vi "Actor Core.vi"(8 "error in":errorcluster, 11 "Timed Loop Controller":refnum<class "Timed Loop Controller.lvclass">) -> (0 "error out":errorcluster, 3 "Actor out":refnum<class "Actor.lvclass">)   [LabVIEW 2016, in "Timed Loop Controller.lvlib" / "Timed Loop Controller.lvclass"]
doc: "This is Actor Core.vi, the main message handling loop for Actors. An actor usually just sits in this loop and processes messages as they arrive. Any error returned by the message Do.vi call will stop the loop, with error code 43 as the cannonical signal to stop with no error sent to caller. Descendants may override that in Handle Error.vi."
uses:
  Timed Loop Controller.lvclass
  C:/Program Files (x86)/National Instruments/LabVIEW 2016/vi.lib/ActorFramework/Actor/Actor.lvclass
  <vilib>/ActorFramework/Actor/Actor.lvclass
  <vilib>/ActorFramework/Actor/Actor.lvclass/Actor.ctl
  <vilib>/ActorFramework/Message Enqueuer/Message Enqueuer.lvclass/Message Enqueuer.ctl
  Timed Loop Controller.lvclass/Timed Loop Controller.ctl
  <vilib>/ActorFramework/Message Enqueuer/Init from Existing Queue.vi
  <vilib>/ActorFramework/Message Enqueuer/Enqueue.vi
  Timed Loop Controller Messages/Update Msg/Update Msg.lvclass
  C:/Program Files (x86)/National Instruments/LabVIEW 2016/vi.lib/ActorFramework/Message/Message.lvclass
  <vilib>/Utility/LVClass/Get LV Class Name.vi
  <resource>/AFDebug/Generate Trace for Message.vi
  <vilib>/ActorFramework/Message Priority Queue/Priority Enqueue.vi
  Controller Actor/Controller Actor.lvclass
  <vilib>/ActorFramework/Message Enqueuer/Message Enqueuer.lvclass
panel:
  in  "stop?":bool
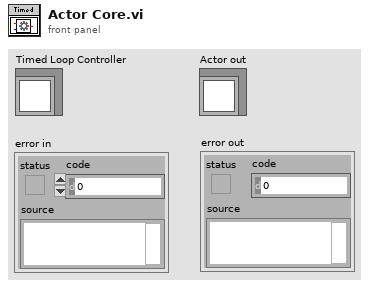
[diagram p1: front panel]
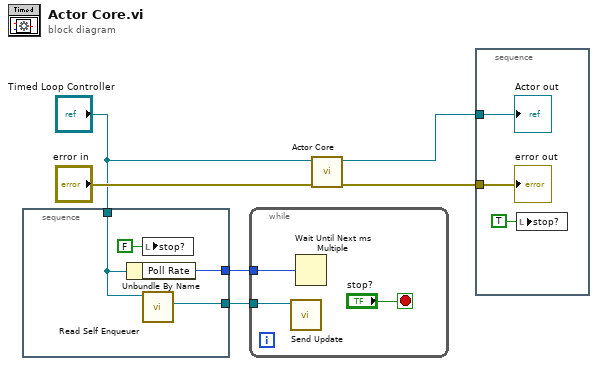
[diagram p0: block diagram]
diagram:
  n1 = stacked-sequence {
    tunnel: "Timed Loop Controller" -> [w10]
    tunnel: [w9] -> w2
    tunnel: [w8] -> w1
    frame #0 {
      n2 = Unbundle By Name(w10) -> ("Poll Rate"=w9:u32)
      n3 = local write "stop?"(FALSE) -> ()
      n4 = call <vilib>:"Read Self Enqueuer.vi"("Actor"=w10) -> ("Self Enqueuer"=w8:refnum<class "Message Enqueuer.lvclass">)  [unwired: 10 in]
    }
  }
  n5 = while {
    tunnel: w1 -> [w13]
    tunnel: w2 -> [w11]
    stop <- "stop?" stop-if-true
    n6 = call "Send Update.vi"("Message Enqueuer in"=w13) -> ()  [unwired: 9 in, 2 out]
    n7 = Wait Until Next ms Multiple(millisecond multiple=w11) -> ()  [unwired: 1 out]
  }
  n8 = call-parent "Actor Core.vi"("error in"="error in", "Event Source in"="Timed Loop Controller") -> ("error out"=w6:errorcluster, "Event Source out"=w3:refnum<class "Actor.lvclass">)  [unwired: 8 in]
  n9 = stacked-sequence {
    tunnel: w6 -> [w16]
    tunnel: w3 -> [w15]
    frame #0 {
      n10 = local write "stop?"(TRUE) -> ()
      "error out" <- w16
      "Actor out" <- w15
    }
  }
